vi "Real LU Linear Equations.vi"(2 "Known Vector":dbl[](array[numeric]) format="%.2f", 3 "LU Info":cluster{"LU":dbl[][], "Pivot":i32[]} {"LU" format="%.3f"}) -> (0 "error":i32, 1 "Solution Vector":dbl[](array[numeric]) format="%.2f")   [LabVIEW 2010, in "NI_AALBase.lvlib"]
doc: "Solves a linear system of simultaneous equations, if possible. The system is solved using the method known as L-U decomposition."
uses:
  NI_AALBase.lvlib
  lvanlys.dll
panel:
  # "Real LU Linear Equations"
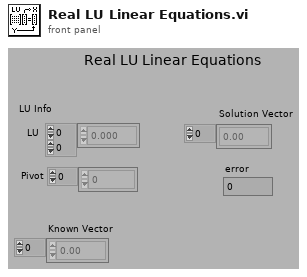
[diagram p1: front panel]
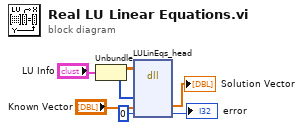
[diagram p0: block diagram]
diagram:
  n1 = Unbundle("LU Info") -> ("LU"=w6:dbl[][], "Pivot"=w5:i32[])
  n2 = dll-call lib="C:/Program Files/National Instruments/LabVIEW 2010/resource/lvanlys.*" fn="LULinEqs_head"("LU"=w6, "Pivot"=w5, "Known Vector"="Known Vector", "error"=0) -> ("Known Vector"=→"Solution Vector":dbl[], "error"=→"error":i32)  [unwired: 6 in, 2 out]
